vi "Window Properties by Name.vi"(9 "window parameter":dbl=nan, 10 "window":T1 items=["Rectangle"=0, "Hanning"=1, "Hamming"=2, "Blackman-Harris"=3, "Exact Blackman"=4, "Blackman"=5, "Flat Top"=6, "4 Term B-Harris "=7, "7 Term B-Harris"=8, "Low Sidelobe"=9, "Blackman Nuttall"=11, "Triangle"=30, "Bartlett-Hanning"=31, "Bohman"=32, "Parzen"=33, "Welch"=34, "Kaiser"=60, "Dolph-Chebyshev"=61, "Gaussian"=62], 11 "size":i32) -> (0 "error":i32, 2 "coherent gain":dbl, 3 "eq noise BW":dbl)   [LabVIEW 2010, in "NI_AALPro.lvlib"]
doc: "Computes the coherent gain and equivalent noise bandwidth of a window. You must manually select the polymorphic instance you want to use."
uses:
  NI_AALPro.lvlib
  windowTd.ctl
  lvanlys.dll
panel:
  # "Window Properties"
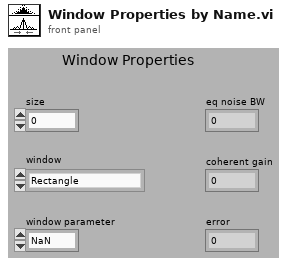
[diagram p1: front panel]
types:
  T1 = typedef "NI_AALPro.lvlib/windowTd.ctl" = u32
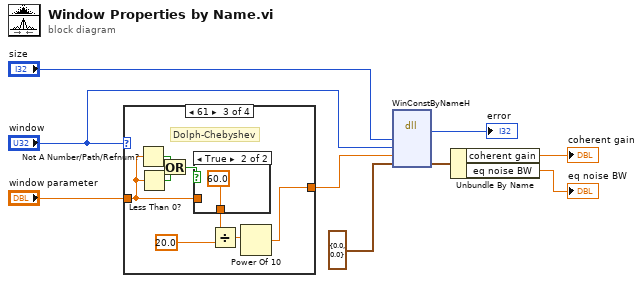
[diagram p0: block diagram]
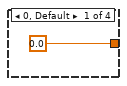
[diagram p2: hidden frame]
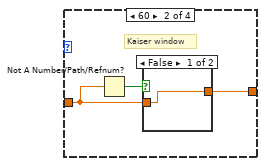
[diagram p3: hidden frame]
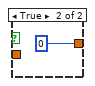
[diagram p4: hidden frame]
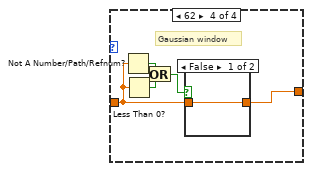
[diagram p6: hidden frame]
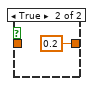
[diagram p7: hidden frame]
diagram:
  n1 = case shown="61" "window" {
    tunnel: [0.0 ("s(db)") w13 w21 w30] -> w2
    tunnel: "window parameter" -> [_ w12 w19 w28]
    frame 0, Default {
    }
    frame 60 {
      # "Kaiser window"
      n2 = Not A Number/Path/Refnum?(number/path/refnum=w12) -> (NaN/Path/Refnum?=w11:bool)
      n3 = case shown="False" w11 {
        tunnel: [w14 0] -> w13
        tunnel: w12 -> [w14 _]
        frame False {
        }
        frame True {
        }
      }
    }
    frame 61 {
      # "Dolph-Chebyshev"
      n4 = Not A Number/Path/Refnum?(number/path/refnum=w19) -> (NaN/Path/Refnum?=w18:bool)
      n5 = Less Than 0?(x=w19) -> (x < 0?=w17:bool)
      n6 = Or(x=w18, y=w17) -> (x .or. y?=w16:bool)
      n7 = case shown="True" w16 {
        tunnel: [w24 60.0 ("y")] -> w20
        tunnel: w19 -> [w24 _]
        frame False {
        }
        frame True {
        }
      }
      n8 = Divide(x=w20, y=20.0) -> (x/y=w22:dbl)
      n9 = Power Of 10(x=w22) -> (10^x=w21:dbl)
    }
    frame 62 {
      # "Gaussian window"
      n10 = Not A Number/Path/Refnum?(number/path/refnum=w28) -> (NaN/Path/Refnum?=w29:bool)
      n11 = Less Than 0?(x=w28) -> (x < 0?=w27:bool)
      n12 = Or(x=w29, y=w27) -> (x .or. y?=w26:bool)
      n13 = case shown="False" w26 {
        tunnel: w28 -> [w31 _]
        tunnel: [w31 0.2 ("para")] -> w30
        frame False {
        }
        frame True {
        }
      }
    }
  }
  n14 = dll-call lib="C:/Program Files/National Instruments/LabVIEW 2010/resource/lvanlys.*" fn="WinConstByNameH"("size"="size", "winType"="window", "winParameter"=w2, "winConst"=cluster{"eq noise BW":dbl, "coherent gain":dbl} {"eq noise BW"=0.0, "coherent gain"=0.0} ("window constants")) -> ("return type"=→"error":i32, "winConst"=w5:cluster{"eq noise BW":dbl, "coherent gain":dbl})  [unwired: 6 in, 2 out]
  n15 = Unbundle By Name(w5) -> ("coherent gain"=→"coherent gain":dbl, "eq noise BW"=→"eq noise BW":dbl)
